vi "Acquisition_analogique.vi"() -> (1 "Température":dbl, 2 "Girouette":dbl, 3 "Humidité":dbl, 4 "Lumière":dbl)   [LabVIEW 2017]
uses:
  <vilib>/DAQmx/read.llb/DAQmx Read (Analog 1D DBL NChan 1Samp).vi
  <vilib>/DAQmx/create/channels.llb/DAQmx Create Channel (AI-Voltage-Basic).vi
  <vilib>/DAQmx/miscellaneous.llb/DAQmx Fill In Error Info.vi
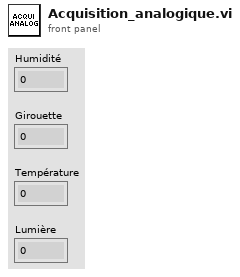
[diagram p1: front panel]
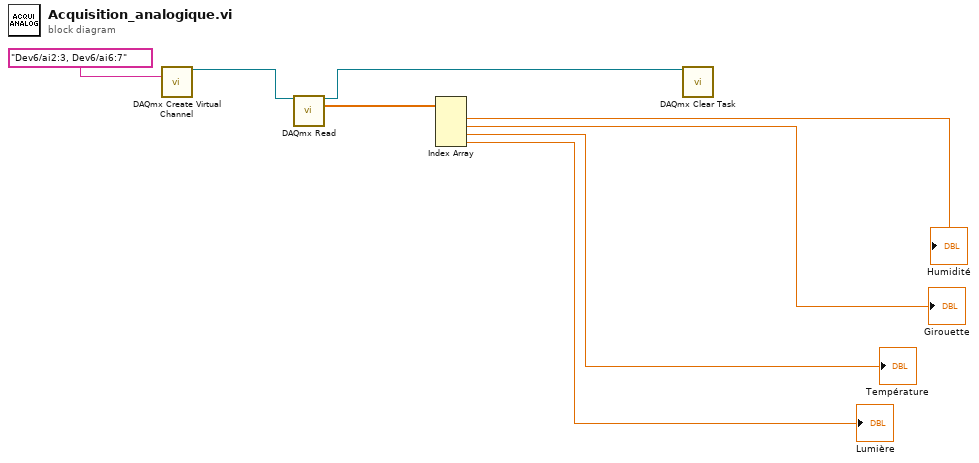
[diagram p0: block diagram]
diagram:
  n1 = call-poly <vilib>:"DAQmx Create Virtual Channel.vi"("physical channels"=tag "Dev6/ai2:3, Dev6/ai6:7") -> ("task out"=w5:refnum<k21>)  [unwired: 13 in, 1 out]
  n2 = call-poly <vilib>:"DAQmx Read.vi"("task/channels in"=w5) -> ("task out"=w7:refnum<k21>, "data"=w6:dbl[])  [unwired: 12 in, 1 out]
  n3 = Index Array(array=w6) -> (element #1=→"Humidité":dbl, element #2=→"Girouette":dbl, element #3=→"Température":dbl, element #4=→"Lumière":dbl)  [unwired: 4 in]
  n4 = call <vilib>:"DAQmx Clear Task.vi"("task in"=w7) -> ()  [unwired: 14 in, 1 out]
